vi "Initialize Control.vi"(8 "error in (no error)":errorcluster, 11 "ScrollZoomGraphChart in":refnum<class "ScrollZoomGraphChart.lvclass">) -> (0 "error out":errorcluster, 3 "ScrollZoomGraphChart out":refnum<class "ScrollZoomGraphChart.lvclass">)   [LabVIEW 2025, in "ScrollZoomGraphChart.lvclass"]
doc: "The <b>Initialize VI</b> is a dynamic dispatch VI that must be overwritten in every QControl Class. It must <b>Call Parent Method</b> so that it recursively calls the initialize routine all of the way up the inheritance hierarchy. \n\nThe top most call is to the <b>Initialize Control VI</b> in Control.lvclass. This is the VI that starts the <b>Event Handler VI</b> if there was one overwritten in the QControl.\n<b> </b> <b> </b>\n©2016 Q Software Innovations, LLC (QSI)\nwritten by Quentin Alldredge\nproduced in LabVIEW 2015\n\nsupport@qsoftwareinnovations.com\nwww.qsoftwareinnovations.com\n\nAll rights reserved.\n\nRedistribution and use in source and binary forms, with or without modification, are permitted provided that the following conditions are met:\n\n * Redistributions of source code must retain the above copyright notice, this list of conditions and the following disclaimer.\n * Redistributions in binary form must reproduce the above copyright notice, this list of conditions and the following disclaimer in the documentation and/or other materials provided with the distribution.\n * Neither the name of Q Software Innovations, LLC. nor the names of its contributors may be used to endorse or promote products derived from this software without specific prior written permission.\n\nTHIS SOFTWARE IS PROVIDED BY THE COPYRIGHT HOLDERS AND CONTRIBUTORS \"AS IS\" AND ANY EXPRESS OR IMPLIED WARRANTIES, INCLUDING, BUT NOT LIMITED TO, THE IMPLIED WARRANTIES OF MERCHANTABILITY AND FITNESS FOR A PARTICULAR PURPOSE ARE DISCLAIMED. IN NO EVENT SHALL THE COPYRIGHT OWNER OR CONTRIBUTORS BE LIABLE FOR ANY DIRECT, INDIRECT, INCIDENTAL, SPECIAL, EXEMPLARY, OR CONSEQUENTIAL DAMAGES (INCLUDING, BUT NOT LIMITED TO, PROCUREMENT OF SUBSTITUTE GOODS OR SERVICES; LOSS OF USE, DATA, OR PROFITS; OR BUSINESS INTERRUPTION) HOWEVER CAUSED AND ON ANY THEORY OF LIABILITY, WHETHER IN CONTRACT, STRICT LIABILITY, OR TORT (INCLUDING NEGLIGENCE OR OTHERWISE) ARISING IN ANY WAY OUT OF THE USE OF THIS SOFTWARE, EVEN IF ADVISED OF THE POSSIBILITY OF SUCH DAMAGE."
uses:
  ScrollZoomGraphChart.lvclass
  ScrollZoomGraphChart.lvclass/ScrollZoomGraphChart.ctl
  <vilib>/QSI/QControls/QControl Classes/GraphChart/GraphChart.lvclass
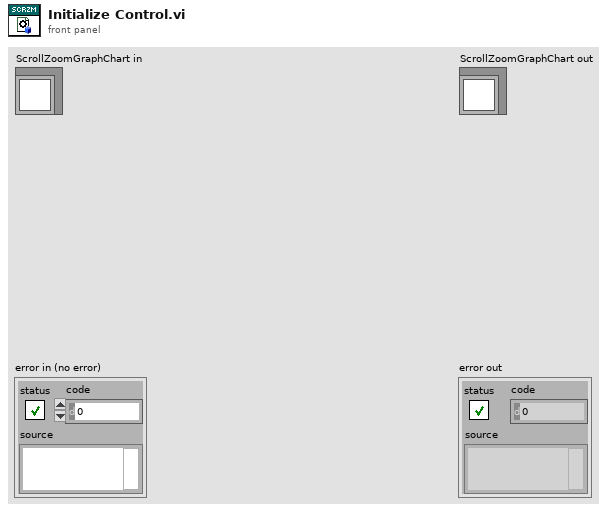
[diagram p1: front panel]
types:
  T1 = typedef "ScrollZoomGraphChart.lvclass/State Data.ctl" = cluster{"X Scales":refnum<vi>[], "Y Scales":refnum<vi>[], "Owning VI":refnum<vi>}
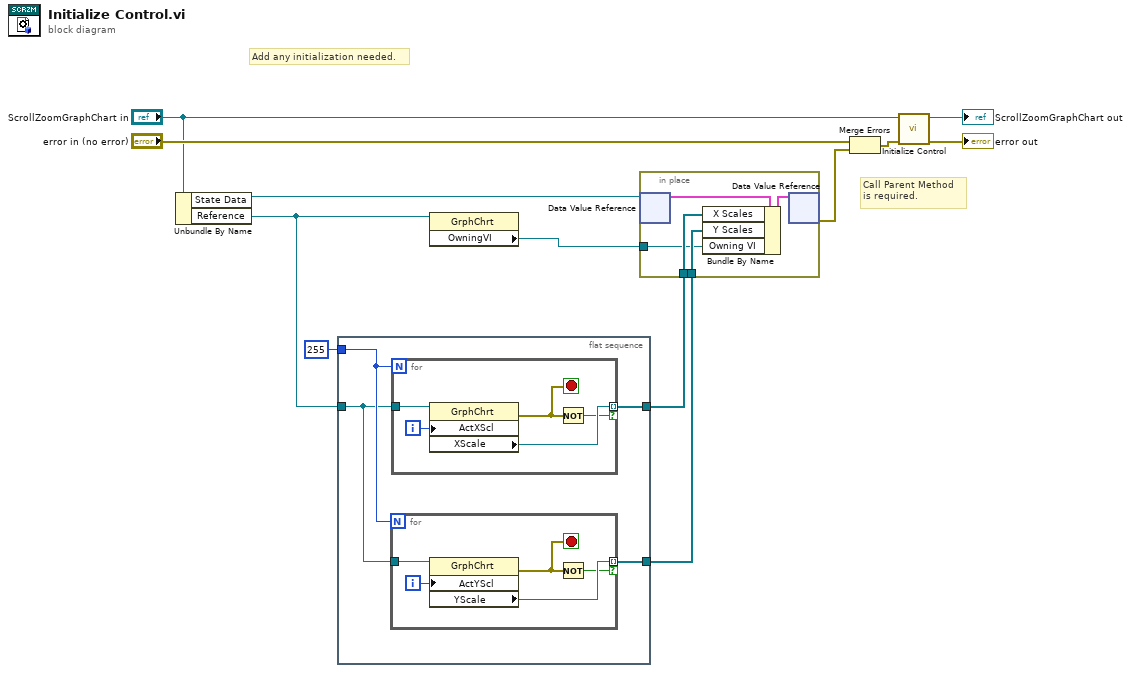
[diagram p0: block diagram]
diagram:
  # "Add any initialization needed."
  # "Call Parent Method\nis required."
  n1 = Unbundle By Name("ScrollZoomGraphChart in") -> ("State Data"=w8:refnum<data-value>, "Reference"=w2:refnum<vi>)
  n2 = flat-sequence {
    tunnel: [w16] -> w6
    tunnel: [w15] -> w5
    tunnel: 255 -> [w14]
    tunnel: w2 -> [w13]
    frame #0 {
      n3 = for {
        N: w14 -> [_]
        tunnel: w13 -> [w26]
        tunnel: [w24] -> w15 mode=indexing if=w22
        i -> [w25]
        stop <- w23 stop-if-true
        n4 = property class="GrphChrt"(reference=w26, "ActYScl"=w25) -> (error out=w23:errorcluster, "YScale"=w24:refnum<vi>)  [unwired: 1 in, 1 out]
        n5 = Not(x=w23) -> (.not. x?=w22:bool)
      }
      n6 = for {
        N: w14 -> [_]
        tunnel: w13 -> [w21]
        tunnel: [w19] -> w16 mode=indexing if=w17
        i -> [w20]
        stop <- w18 stop-if-true
        n7 = property class="GrphChrt"(reference=w21, "ActXScl"=w20) -> (error out=w18:errorcluster, "XScale"=w19:refnum<vi>)  [unwired: 1 in, 1 out]
        n8 = Not(x=w18) -> (.not. x?=w17:bool)
      }
    }
  }
  n9 = property class="GrphChrt"(reference=w2) -> ("OwningVI"=w1:refnum<vi>)  [unwired: 1 in, 2 out]
  n10 = in-place {
    in-place-border: w6 -> [w29]
    in-place-border: w5 -> [w28]
    in-place-border: w1 -> [w27]
    n11 = in-place-dvr #1(w8) -> (w31:T1)  [unwired: 1 out]
    n12 = Bundle By Name(cluster=w31, "X Scales"=w29, "Y Scales"=w28, "Owning VI"=w27) -> (w30:T1)
    n13 = in-place-dvr #1(w30) -> (w3:errorcluster)  [unwired: 1 out]
  }
  n14 = Merge Errors("error in (no error)", w3) -> (w4:errorcluster)
  n15 = call-parent "Initialize Control.vi"("error in (no error)"=w4, "Control in"="ScrollZoomGraphChart in") -> ("error out"=→"error out":errorcluster, "Control out"=→"ScrollZoomGraphChart out":refnum<class "ScrollZoomGraphChart.lvclass">)  [unwired: 8 in]
